vi "Time2Samples.vi"(0 "Duration (ms)":dbl, 1 "Sampling rate (Hz)":dbl) -> (2 "Samples":i32)   [LabVIEW 2015]
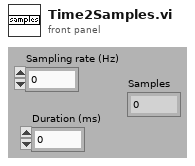
[diagram p1: front panel]
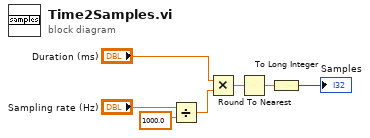
[diagram p0: block diagram]
diagram:
  n1 = Divide(x="Sampling rate (Hz)", y=1000.0) -> (x/y=w6:dbl)
  n2 = Multiply(x="Duration (ms)", y=w6) -> (x*y=w4:dbl)
  n3 = Round To Nearest(number=w4) -> (nearest integer value=w3:dbl)
  n4 = To Long Integer(number=w3) -> (32bit integer=→"Samples":i32)
